vi "RT_MPU Init.vi"(8 "error in":errorcluster, 11 "FPGA VI Reference In":T1) -> (0 "error out":errorcluster, 3 "FPGA VI Reference Out":T1)   [LabVIEW 2018]
uses:
  Data Def/RT_FPGA VI Reference.ctl
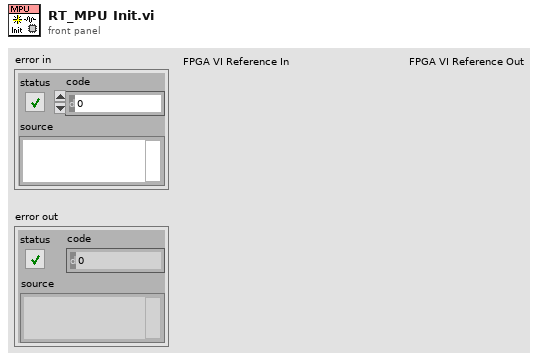
[diagram p1: front panel]
types:
  T1 = typedef "RT_FPGA VI Reference.ctl" = refnum<k20>
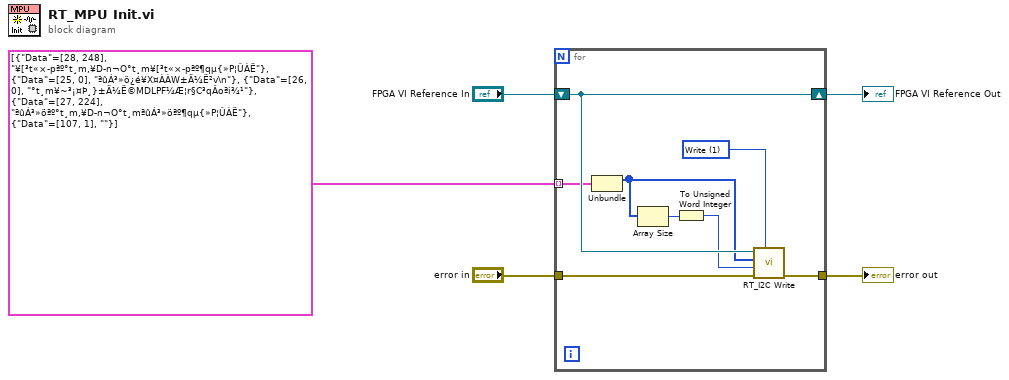
[diagram p0: block diagram]
diagram:
  n1 = for {
    tunnel: "error in" -> [w13]
    tunnel: [w12] -> w4
    shift-right: [w11] -> w2
    shift-left: "FPGA VI Reference In" -> [w11]
    tunnel: cluster{"Data":u8[], string}[] [{"Data"=[28, 248], "¥[³t«×­pªº°t¸m,¥D­n¬O°t¸m¥[³t«×­pªº¶qµ{»P¦ÛÀË"}, {"Data"=[25, 0], "ªûÁ³»ö¿é¥X¤ÀÀW±Ä¼Ë²v\n"}, {"Data"=[26, 0], "°t¸m¥~³¡¤Þ¸}±Ä¼Ë©MDLPF¼Æ¦r§C³qÂoªi¾¹"}, {"Data"=[27, 224], "ªûÁ³»öªº°t¸m,¥D­n¬O°t¸mªûÁ³»öªº¶qµ{»P¦ÛÀË"}, {"Data"=[107, 1], ""}] -> [w10] mode=indexing
    w6 = u8 1 items=["Write & Read", "Write", "Read"] ("Command (Write & Read)")
    n2 = Unbundle(w10) -> ("Data"=w9:u8[])  [unwired: 1 out]
    n3 = Array Size(array=w9) -> (size(s)=w8:i32)
    n4 = To Unsigned Word Integer(number=w8) -> (unsigned 16bit integer=w7:u16)
    n5 = call "RT_I2C Write.vi"("Command (Write & Read)"=w6, "error in"=w13, "Number of Bytes to Write"=w7, "Data"=w9, "FPGA VI Reference In"=w11) -> ("error out"=w12:errorcluster)  [unwired: 5 in, 1 out]
  }
  "error out" <- w4
  "FPGA VI Reference Out" <- w2
